vi "Connect LocalQueue.vi"(6 "timeout (500 ms)":i32=500, 8 "error in (no error)":errorcluster, 11 "Queue Name":string) -> (0 "error out":errorcluster, 3 "LocalQueueConnection":refnum<class "LocalQueueConnection.lvclass">)   [LabVIEW 2013, in "MQTT_Queue.lvlib" / "LocalQueueConnection.lvclass"]
uses:
  LocalQueueConnection.lvclass
  <vilib>/LabVIEW Open Source Project/MQTT Connection/MQTT_Connection/Connection/Connection.lvclass
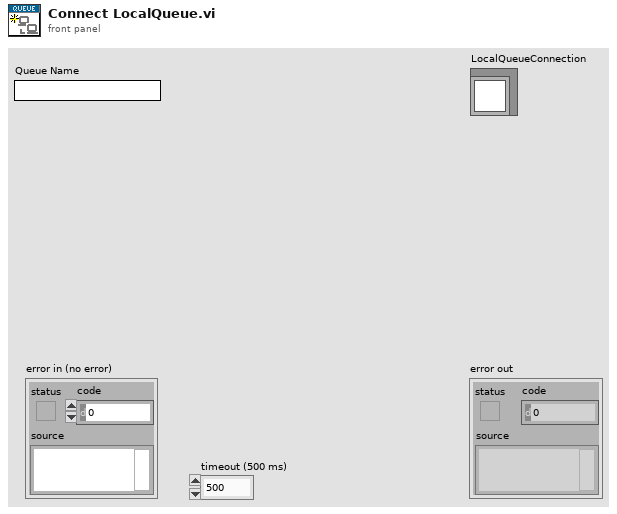
[diagram p1: front panel]
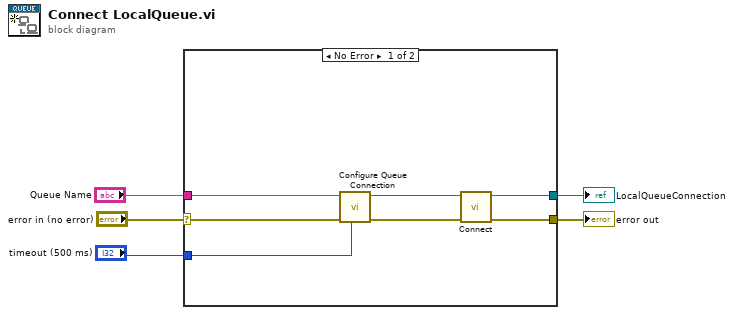
[diagram p0: block diagram]
diagram:
  n1 = case shown="No Error" "error in (no error)" {
    selector: "error in (no error)" -> [w9 w13]
    tunnel: [w11 w13] -> w4
    tunnel: [w12 _] -> w3
    tunnel: "Queue Name" -> [w7 _]
    tunnel: "timeout (500 ms)" -> [w6 _]
    frame No Error {
      n2 = call "Configure Queue Connection.vi"("timeout (500 ms)"=w6, "error in (no error)"=w9, "Queue Name"=w7) -> ("error out"=w8:errorcluster, "LocalQueueConnection"=w10:refnum<class "LocalQueueConnection.lvclass">)  [unwired: 7 in]
      n3 = call <vilib>:"Connect.vi"("error in (no error)"=w8, "Connection in"=w10) -> ("error out"=w11:errorcluster, "Connection out"=w12:refnum<class "LocalQueueConnection.lvclass">)  [unwired: 8 in]
    }
    frame Error {
    }
  }
  "error out" <- w4
  "LocalQueueConnection" <- w3
